vi "CSConnect.destructor.vi"(0 "i ref in":refnum<vi>, 5 "error in (no error)":errorcluster) -> (19 "error out":errorcluster)   [LabVIEW 2014, in "CSConnect.lvlib"]
doc: "This is the destructor of a class.\n\nLicense Agreement for this software:\n\nCopyright (C)\nGesellschaft für Schwerionenforschung, GSI\nPlanckstr. 1\n64291 Darmstadt\nGermany\n\nContact: D.Beck@gsi.de \n\nThis program is free software; you can redistribute it and/or modify it under the terms of the \nGNU General Public License as published by the Free Software Foundation; either version 2 of \nthe license, or (at your option) any later version.\n\nThis program is distributed in the hope that it will be useful, but WITHOUT ANY WARRANTY; \nwithout even the implied warranty of MERCHANTABILITY or FITNESS FOR A PARTICULAR PURPOSE. See the GNU General License for more details (http://www.gnu.org).\n\nGesellschaft für Schwerionenforschung, GSI\nPlanckstr. 1, 64291 Darmstadt, Germany\nFor all questions and ideas contact: M.Richter@gsi.de, H.Brand@gsi.de or D.Beck@gsi.de.\nLast update: 16-JUN-2004"
uses:
  CSConnect.lvlib
  CS_Core/CSApplicationBaseClasses/PSChannelBase/PSChannelBase.lvlib
  CSlibraries-extern/DimLVEvent/LVDimInterface/LVDimInterface.lvlib
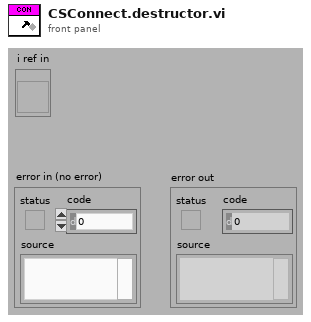
[diagram p1: front panel]
types:
  T1 = typedef "CSConnect.lvlib/CSConnect.i attribute.ctl" = cluster{"In-Array":cluster{"Alias":string, "Value":dbl, "neededOuts":bool[]}[], "Out-Array":cluster{"ObjectName":string, "VoltFunctionName":string, "OnOffFunctionName":string, "Channel":string, "Calculation-Formula":string}[], "OutChannelsID":i32, "InOutMatrixID":i32}
  T2 = enum16{"SetAttribute", "GetAttribute", "CreateAttribute", "DestroyAttribute", "DestroyAllAtributes"}
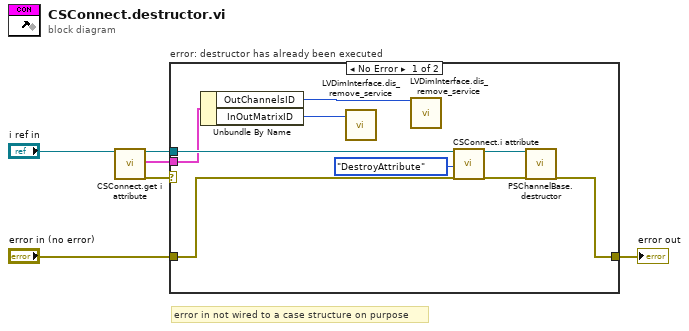
[diagram p0: block diagram]
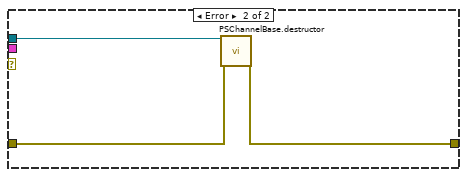
[diagram p2: hidden frame]
diagram:
  # "error in not wired to a case structure on purpose"
  n1 = call "CSConnect.get i attribute.vi"("i ref in"="i ref in") -> ("i ref out"=w2:refnum<vi>, "i attribute"=w1:T1, "error out"=w3:errorcluster)  [unwired: 16 in]
  n2 = case "error: destructor has already been executed" shown="No Error" w3 {
    tunnel: [w12 w16] -> w6
    tunnel: "error in (no error)" -> [w11 w17]
    tunnel: w2 -> [w10 w18]
    tunnel: w1 -> [w9 _]
    frame No Error {
      n3 = Unbundle By Name(w9) -> ("OutChannelsID"=w8:i32, "InOutMatrixID"=w7:i32)
      n4 = call "LVDimInterface.dis_remove_service.vi"("my_serviceID"=w7) -> ()  [unwired: 18 in, 1 out]
      n5 = call "LVDimInterface.dis_remove_service.vi"("my_serviceID"=w8) -> ()  [unwired: 18 in, 1 out]
      n6 = call "CSConnect.i attribute.vi"("VI Refnum"=w10, "Action"=T2."DestroyAttribute", "error in (no error)"=w11) -> ("VI Refnum out"=w14:refnum<vi>, "error out"=w13:errorcluster)  [unwired: 14 in, 1 out]
      n7 = call "PSChannelBase.destructor.vi"("i ref in"=w14, "error in (no error)"=w13) -> ("error out"=w12:errorcluster)  [unwired: 17 in]
    }
    frame Error {
      n8 = call "PSChannelBase.destructor.vi"("i ref in"=w18, "error in (no error)"=w17) -> ("error out"=w16:errorcluster)  [unwired: 17 in]
    }
  }
  "error out" <- w6
